vi "Tutorial.vi"() -> ()   [LabVIEW 2023]
uses:
  parametertype.ctl
  <vilib>/regexp/Match Regular Expression.xnode
  SECoP.lvlib
panel:
  in  "stop":bool
  out "log 2":string
  out "error out":errorcluster
  in  "stop 2":bool
  in  "DLL path":path=path "D:/shall-repos/SHALL-LabVIEW/64bit"
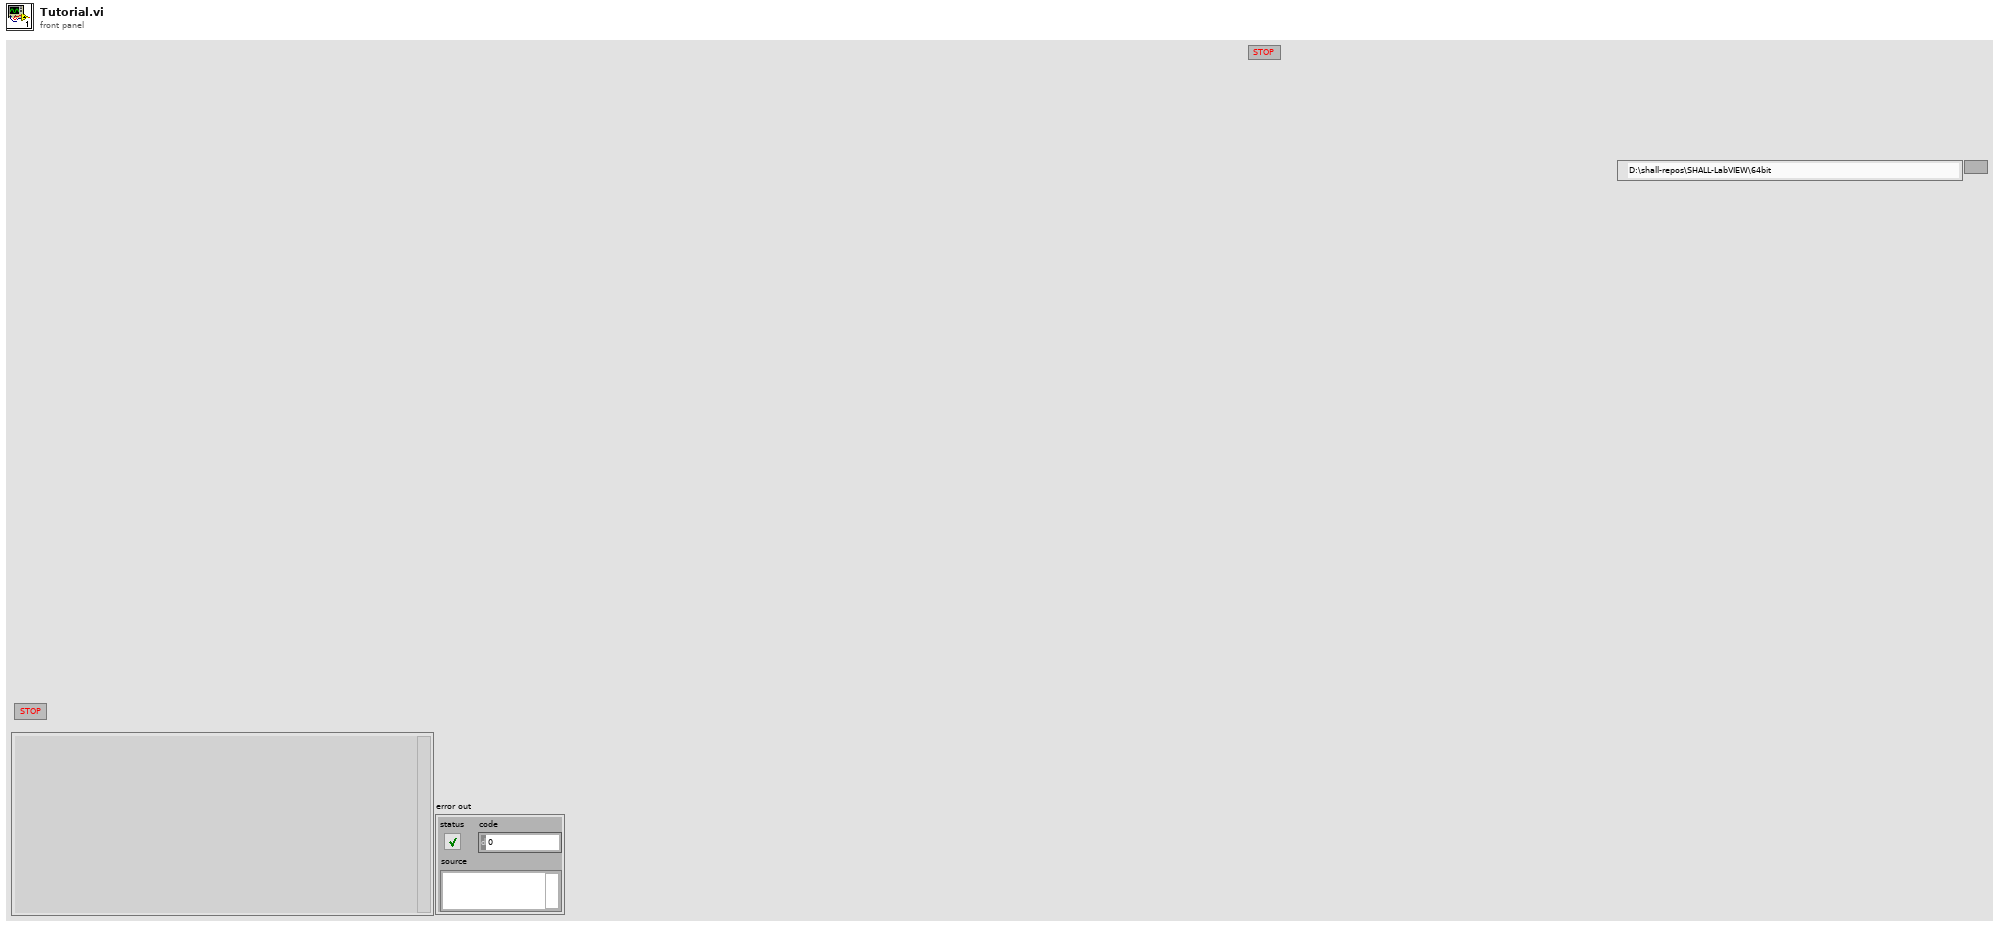
[diagram p1: front panel]
types:
  T1 = typedef "parametertype.ctl" = enum8{"readonly", "readwrite", "command"}
  T2 = cluster{"name":string, "type":T1, "datatype":string, "description":string, dbl}[]
  T3 = typedef "SECoP.lvlib/SECoP-libraries.ctl" = cluster{"serverDLL":path, "variantDLL":path, "cleanup_mode":bool, "Context_ID":string}
  T4 = typedef "SECoP.lvlib/SECoP-action.ctl" = enum32{"any action", "read", "change", "do cmd"}
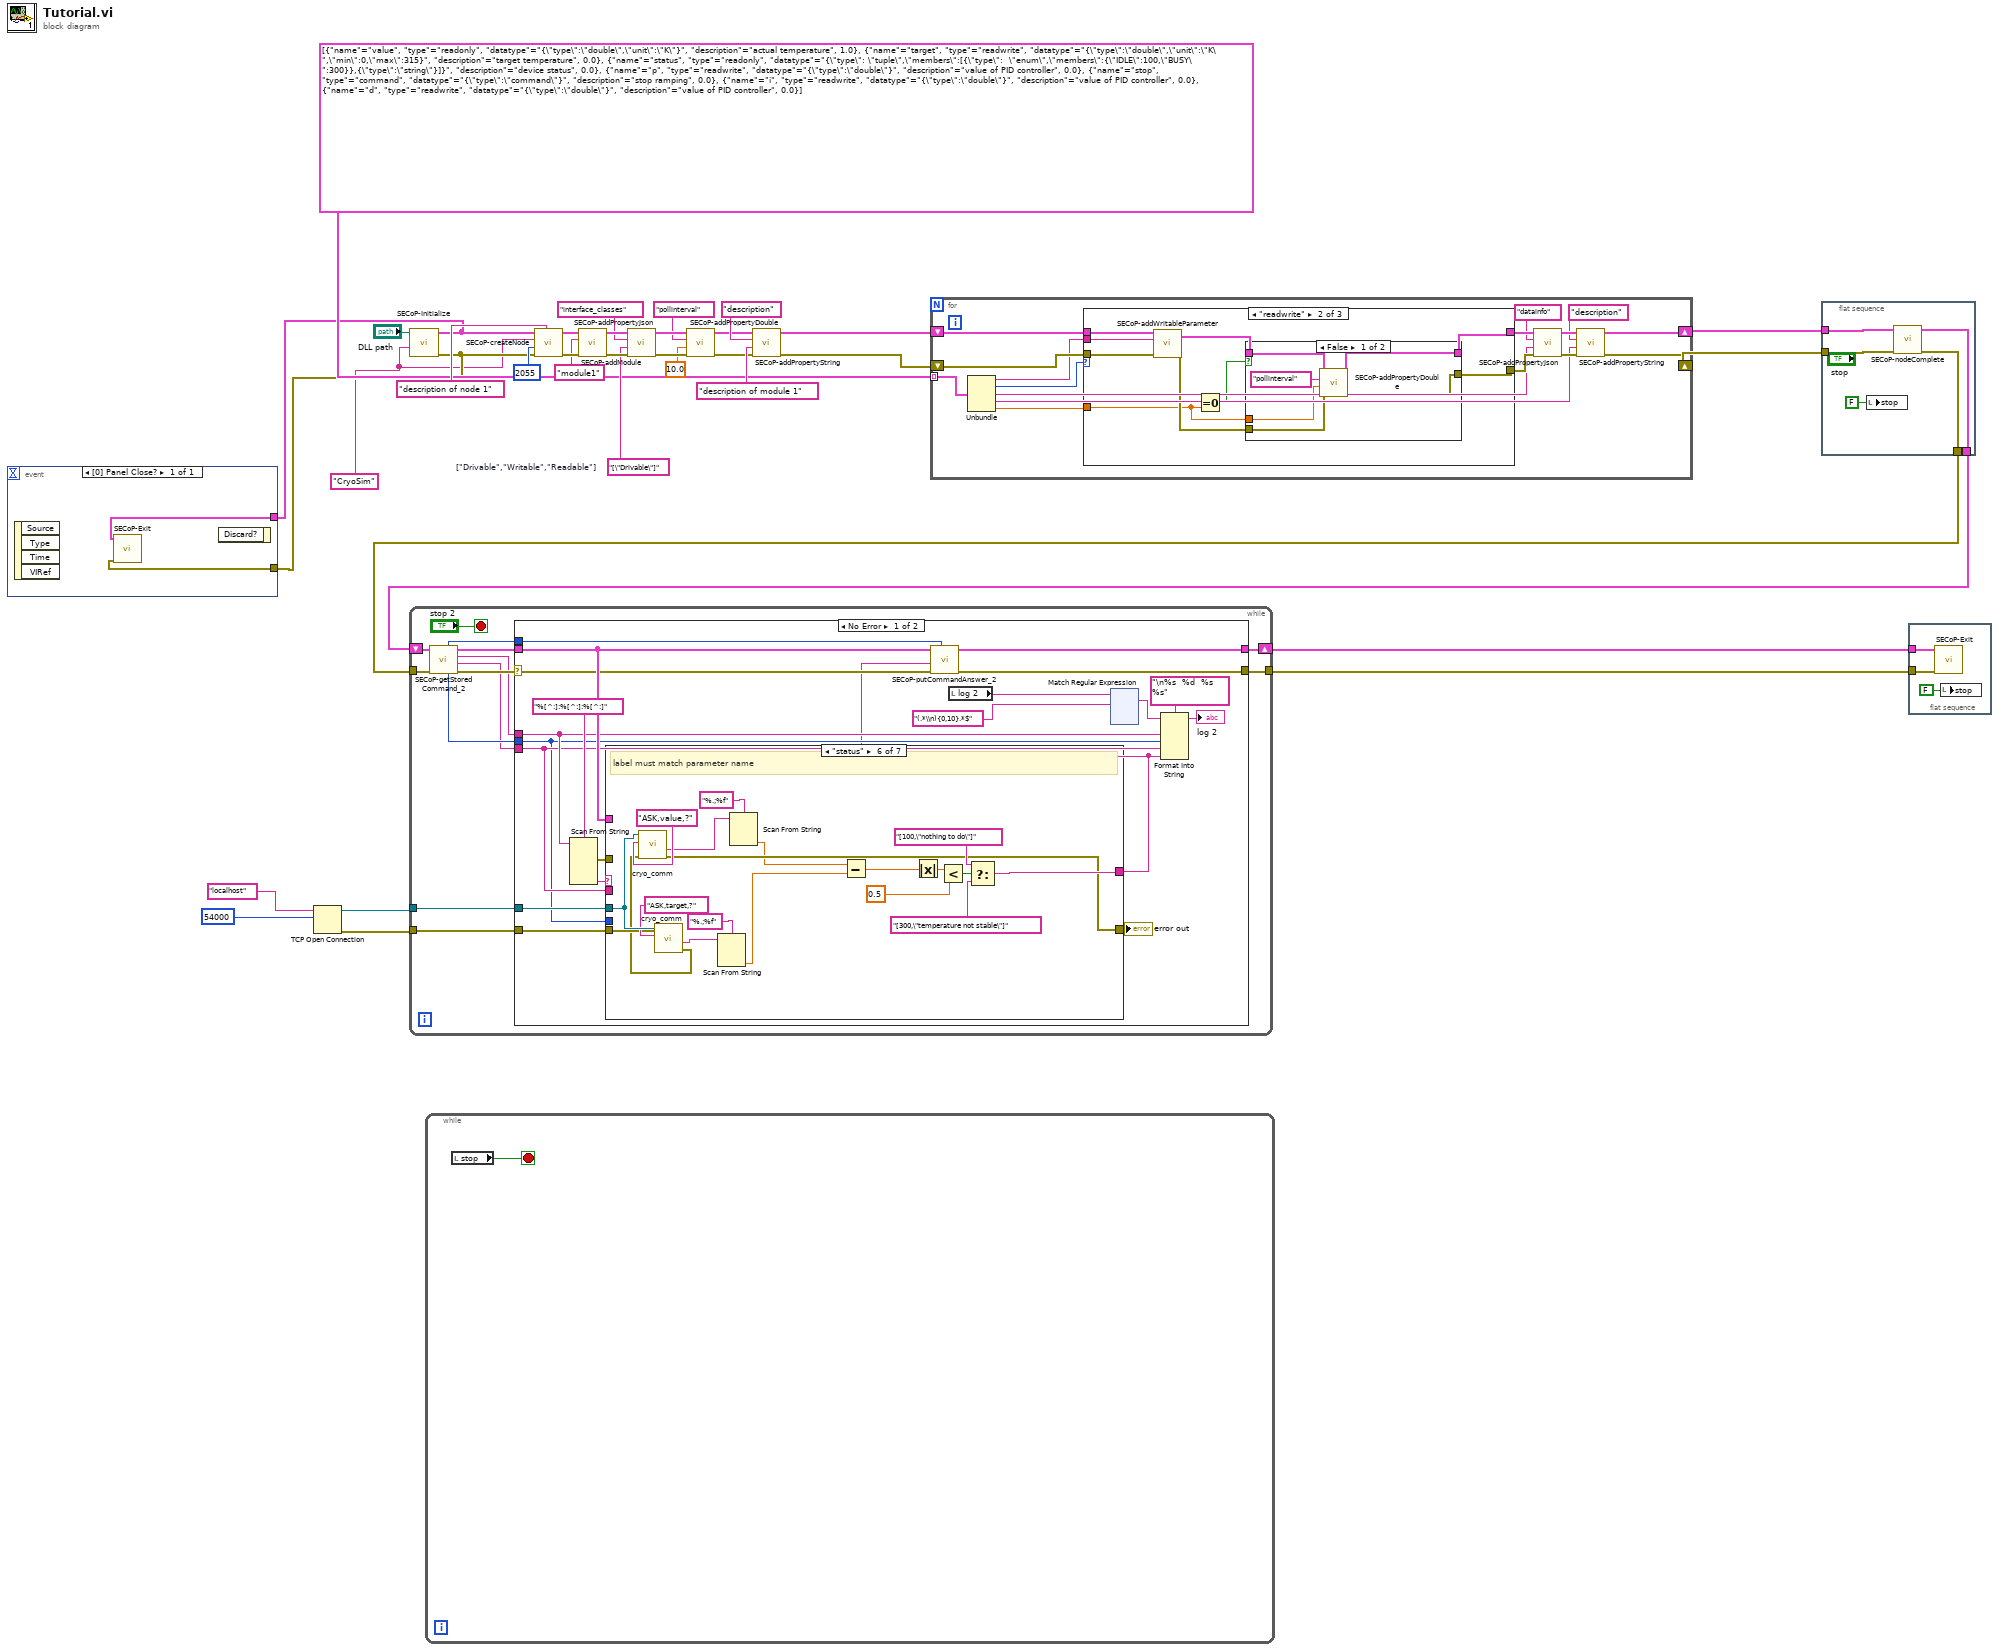
[diagram p0: block diagram]
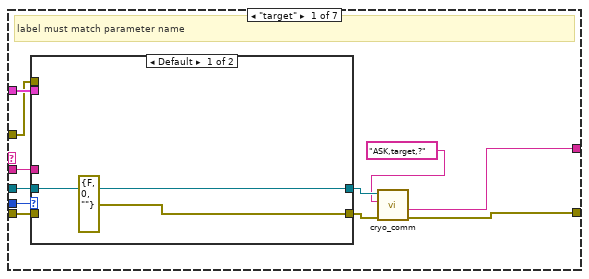
[diagram p2: hidden frame]
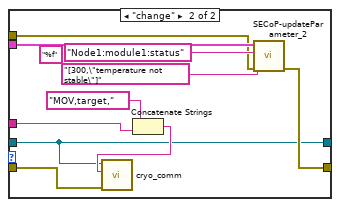
[diagram p3: hidden frame]
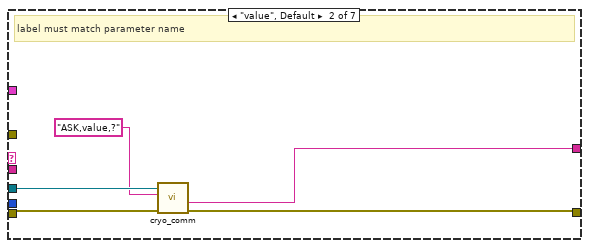
[diagram p4: hidden frame]
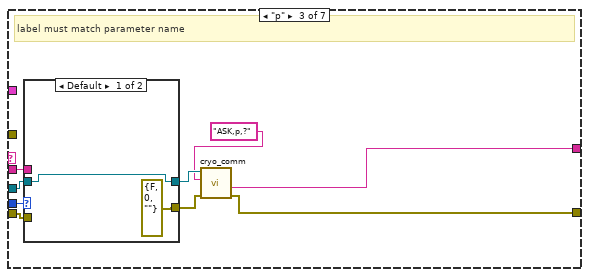
[diagram p5: hidden frame]
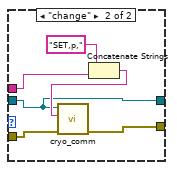
[diagram p6: hidden frame]
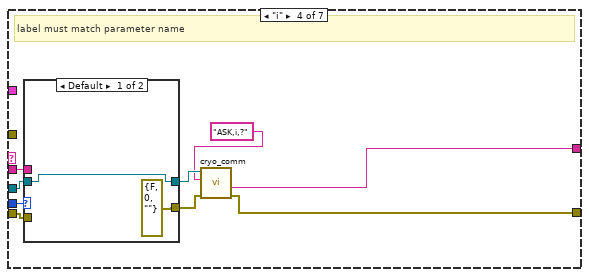
[diagram p7: hidden frame]
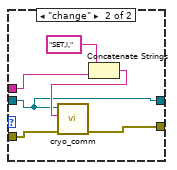
[diagram p8: hidden frame]
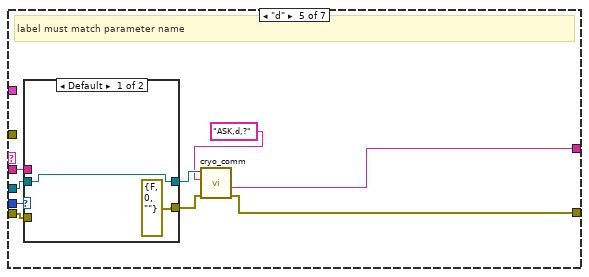
[diagram p9: hidden frame]
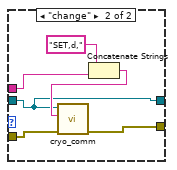
[diagram p10: hidden frame]
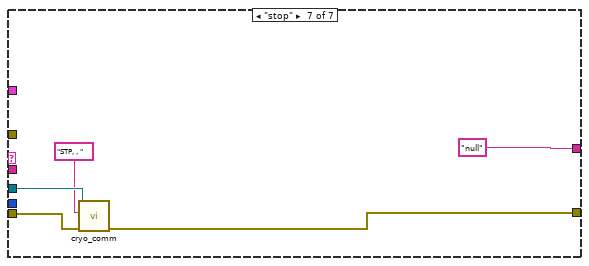
[diagram p11: hidden frame]
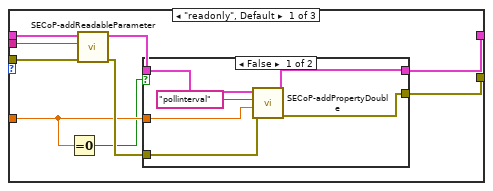
[diagram p13: hidden frame]
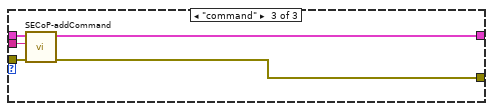
[diagram p16: hidden frame]
diagram:
  w25 = "[\"Drivable\"]"  # ["Drivable","Writable","Readable"]
  w1 = "CryoSim" ("id")
  # "description"
  # "data type as SECoP \"datainfo\""
  # "type"
  # "parameter"
  n1 = TCP Open Connection(address="localhost", remote port or service name=54000) -> (connection ID=w2:refnum<k5>, error out=w3:errorcluster)  [unwired: 3 in]
  n2 = while {
    shift-right: [w47] -> w7
    shift-left: w4 -> [w46]
    tunnel: w5 -> [w45]
    tunnel: [w38] -> w6
    tunnel: w2 -> [w36]
    tunnel: w3 -> [w35]
    stop <- "stop 2" stop-if-true
    n3 = call "SECoP-getStoredCommand_2.vi"("error in (no error)"=w45, "DLL path (in)"=w46) -> ("error out"=w43:errorcluster, "arguments/setvalue"=w39:string, "command/parameter path"=w40:string, "DLL path (out)"=w44:T3, "action"=w41:T4, "command id"=w42:u64)  [unwired: 4 in]
    n4 = case shown="No Error" w43 {
      selector: w43 -> [w66 w288]
      tunnel: w44 -> [w67 w289]
      tunnel: [w65 w289] -> w47
      tunnel: w42 -> [w64 _]
      tunnel: w40 -> [w57 _]
      tunnel: w39 -> [w53 _]
      tunnel: w41 -> [w52 _]
      tunnel: [w63 w288] -> w38
      tunnel: w36 -> [w54 _]
      tunnel: w35 -> [w50 _]
      frame No Error {
        n5 = Scan From String(format string="%[^:]:%[^:]:%[^:]", input string=w57) -> (error out=w56:errorcluster, output 3=w48:string)  [unwired: 7 in, 2 out]
        n6 = case shown="\"status\"" w48 {
          tunnel: [w71 w92 w97 w114 w131 w159 "null"] -> w49
          tunnel: w56 -> [w68 _ _ _ _ _ _]
          tunnel: w54 -> [w77 w93 w103 w120 w137 w158 w169]
          tunnel: w53 -> [w78 _ w102 w119 w136 _ _]
          tunnel: w52 -> [w76 _ w104 w121 w138 _ _]
          tunnel: [w72 w94 w98 w115 w132 w154 w166] -> w51
          tunnel: w50 -> [w75 w95 w101 w118 w135 w155 w168]
          tunnel: w67 -> [w74 _ _ _ _ _ _]
          frame "target" {
            # "label must match parameter name"
            n7 = case shown="Default" w76 {
              tunnel: w78 -> [_ w84]
              tunnel: w77 -> [w80 w82]
              tunnel: [errorcluster {"status"=FALSE, "code"=0, "source"=""} ("error out") w89] -> w73
              tunnel: [w80 w82] -> w70
              tunnel: w75 -> [_ w85]
              tunnel: w74 -> [_ w90]
              tunnel: w68 -> [_ w81]
              frame Default {
              }
              frame "change" {
                (unwired) "%f" ("format string")
                n8 = Concatenate Strings("MOV,target,", w84) -> (w83:string)
                n9 = call "cryo_comm.vi"("error in (no error)"=w85, "String"=w83, "TCP Network Connection in"=w82) -> ()  [unwired: 5 in, 4 out]
                n10 = call "SECoP-updateParameter_2.vi"("error in (no error)"=w81, "value"="[300,\"temperature not stable\"]" ("Value"), "parameter name"="Node1:module1:status" ("Parameter name"), "DLL path (in)"=w90) -> ("error out"=w89:errorcluster)  [unwired: 6 in, 1 out]
              }
            }
            n11 = call "cryo_comm.vi"("error in (no error)"=w73, "String"="ASK,target,?", "TCP Network Connection in"=w70) -> ("error out 2"=w72:errorcluster, "Message [2] (return value)"=w71:string)  [unwired: 5 in, 2 out]
          }
          frame "value", Default {
            # "label must match parameter name"
            n12 = call "cryo_comm.vi"("error in (no error)"=w95, "String"="ASK,value,?", "TCP Network Connection in"=w93) -> ("error out 2"=w94:errorcluster, "Message [2] (return value)"=w92:string)  [unwired: 5 in, 2 out]
          }
          frame "p" {
            # "label must match parameter name"
            n13 = case shown="Default" w104 {
              tunnel: w103 -> [w106 w107]
              tunnel: w102 -> [_ w109]
              tunnel: [w106 w107] -> w99
              tunnel: [errorcluster {"status"=FALSE, "code"=0, "source"=""} ("error out") w111] -> w100
              tunnel: w101 -> [_ w112]
              frame Default {
              }
              frame "change" {
                n14 = Concatenate Strings("SET,p,", w109) -> (w108:string)
                n15 = call "cryo_comm.vi"("error in (no error)"=w112, "String"=w108, "TCP Network Connection in"=w107) -> ("error out 2"=w111:errorcluster)  [unwired: 5 in, 3 out]
              }
            }
            n16 = call "cryo_comm.vi"("error in (no error)"=w100, "String"="ASK,p,?", "TCP Network Connection in"=w99) -> ("error out 2"=w98:errorcluster, "Message [2] (return value)"=w97:string)  [unwired: 5 in, 2 out]
          }
          frame "i" {
            # "label must match parameter name"
            n17 = case shown="Default" w121 {
              tunnel: w120 -> [w123 w124]
              tunnel: w119 -> [_ w126]
              tunnel: [w123 w124] -> w116
              tunnel: [errorcluster {"status"=FALSE, "code"=0, "source"=""} ("error out") w128] -> w117
              tunnel: w118 -> [_ w129]
              frame Default {
              }
              frame "change" {
                n18 = Concatenate Strings("SET,i,", w126) -> (w125:string)
                n19 = call "cryo_comm.vi"("error in (no error)"=w129, "String"=w125, "TCP Network Connection in"=w124) -> ("error out 2"=w128:errorcluster)  [unwired: 5 in, 3 out]
              }
            }
            n20 = call "cryo_comm.vi"("error in (no error)"=w117, "String"="ASK,i,?", "TCP Network Connection in"=w116) -> ("error out 2"=w115:errorcluster, "Message [2] (return value)"=w114:string)  [unwired: 5 in, 2 out]
          }
          frame "d" {
            # "label must match parameter name"
            n21 = case shown="Default" w138 {
              tunnel: w137 -> [w140 w141]
              tunnel: w136 -> [_ w143]
              tunnel: [w140 w141] -> w133
              tunnel: [errorcluster {"status"=FALSE, "code"=0, "source"=""} ("error out") w145] -> w134
              tunnel: w135 -> [_ w146]
              frame Default {
              }
              frame "change" {
                n22 = Concatenate Strings("SET,d,", w143) -> (w142:string)
                n23 = call "cryo_comm.vi"("error in (no error)"=w146, "String"=w142, "TCP Network Connection in"=w141) -> ("error out 2"=w145:errorcluster)  [unwired: 5 in, 3 out]
              }
            }
            n24 = call "cryo_comm.vi"("error in (no error)"=w134, "String"="ASK,d,?", "TCP Network Connection in"=w133) -> ("error out 2"=w132:errorcluster, "Message [2] (return value)"=w131:string)  [unwired: 5 in, 2 out]
          }
          frame "status" {
            # "label must match parameter name"
            n25 = call "cryo_comm.vi"("error in (no error)"=w155, "String"="ASK,target,?", "TCP Network Connection in"=w158) -> ("error out 2"=w153:errorcluster, "Message [2] (return value)"=w152:string)  [unwired: 5 in, 2 out]
            n26 = call "cryo_comm.vi"("error in (no error)"=w153, "String"="ASK,value,?", "TCP Network Connection in"=w158) -> ("error out 2"=w154:errorcluster, "Message [2] (return value)"=w147:string)  [unwired: 5 in, 2 out]
            n27 = Scan From String(format string="%.;%f", input string=w152) -> (output 1=w150:dbl)  [unwired: 3 in, 3 out]
            n28 = Scan From String(format string="%.;%f", input string=w147) -> (output 1=w148:dbl)  [unwired: 3 in, 3 out]
            n29 = Subtract(x=w148, y=w150) -> (x-y=w165:dbl)
            n30 = Absolute Value(x=w165) -> (abs(x)=w164:dbl)
            n31 = Less?(x=w164, y=0.5) -> (x < y?=w162:bool)
            n32 = Select(t="[100,\"nothing to do\"]", s=w162, f="[300,\"temperature not stable\"]") -> (s? t:f=w159:string)
          }
          frame "stop" {
            n33 = call "cryo_comm.vi"("error in (no error)"=w168, "String"="STP, , ", "TCP Network Connection in"=w169) -> ("error out 2"=w166:errorcluster)  [unwired: 5 in, 3 out]
          }
        }
        "error out" <- w51
        n34 = call "SECoP-putCommandAnswer_2.vi"("command id"=w64, "error in (no error)"=w66, "value"=w49, "DLL path (in)"=w67) -> ("error out"=w63:errorcluster, "DLL path (out)"=w65:T3)  [unwired: 6 in]
        n35 = local read "log 2"() -> (w60:string)
        n36 = xnode "Match Regular Expression"("input string"=w60, "regular expression"="(.*\\n){0,10}.*$") -> ("whole match"=w61:string)  [unwired: 4 in, 4 out]
        n37 = Format Into String(format string="\n%s  %d  %s  %s", initial string=w61, w57, w52, w53, w49) -> (resulting string=→"log 2":string)  [unwired: 1 in, 1 out]
      }
      frame Error {
      }
    }
  }
  n38 = call "SECoP-Initialize.vi"("Context ID (in)"=w1, "DLL path (in)"="DLL path") -> ("error out"=w12:errorcluster, "DLL path (out)"=w13:T3)  [unwired: 8 in]
  n39 = event shown="[0] Panel Close?" {
    selector: _ -> [_]
    dyn-events: _ -> [_]
    timeout: _ -> [_]
    tunnel: w13 -> [w291]
    tunnel: w12 -> [w290]
    event Panel Close? {
      n40 = event-data() -> ()  [unwired: 1 in, 4 out]
      n41 = call "SECoP-Exit.vi"("error in (no error)"=w290, "DLL path (in)"=w291) -> ()  [unwired: 9 in, 1 out]
      n42 = event-data() -> ()  [unwired: 2 in, 1 out]
    }
  }
  n43 = while {
    stop <- w292 stop-if-true
    n44 = local read "stop"() -> (w292:bool)
  }
  n45 = call "SECoP-createNode.vi"("description"="description of node 1", "error in (no error)"=w12, "TCP port"=u16 2055, "node id"=w1, "DLL path (in)"=w13) -> ("error out"=w30:errorcluster, "DLL path (out)"=w33:T3)  [unwired: 5 in]
  n46 = call "SECoP-addModule.vi"("error in (no error)"=w30, "module name"="module1" ("name"), "DLL path (in)"=w33) -> ("error out"=w27:errorcluster, "DLL path (out)"=w28:T3)  [unwired: 7 in]
  n47 = call "SECoP-addPropertyJson.vi"("error in (no error)"=w27, "property value"=w25, "property name"="interface_classes" ("name"), "DLL path (in)"=w28) -> ("error out"=w18:errorcluster, "DLL path (out)"=w20:T3)  [unwired: 6 in]
  n48 = call "SECoP-addPropertyDouble.vi"("error in (no error)"=w18, "property value"=10.0, "property name"="pollinterval", "DLL path (in)"=w20) -> ("error out"=w17:errorcluster, "DLL path (out)"=w19:T3)  [unwired: 6 in]
  n49 = call "SECoP-addPropertyString.vi"("error in (no error)"=w17, "property value"="description of module 1" ("name"), "property name"="description" ("name"), "DLL path (in)"=w19) -> ("error out"=w23:errorcluster, "DLL path (out)"=w24:T3)  [unwired: 6 in]
  n50 = for {
    tunnel: T2 [{"name"="value", "type"=enum."readonly", "datatype"="{\"type\":\"double\",\"unit\":\"K\"}", "description"="actual temperature", 1.0}, {"name"="target", "type"=enum."readwrite", "datatype"="{\"type\":\"double\",\"unit\":\"K\",\"min\":0,\"max\":315}", "description"="target temperature", 0.0}, {"name"="status", "type"=enum."readonly", "datatype"="{\"type\": \"tuple\",\"members\":[{\"type\":  \"enum\",\"members\":{\"IDLE\":100,\"BUSY\":300}},{\"type\":\"string\"}]}", "description"="device status", 0.0}, {"name"="p", "type"=enum."readwrite", "datatype"="{\"type\":\"double\"}", "description"="value of PID controller", 0.0}, {"name"="stop", "type"=enum."command", "datatype"="{\"type\":\"command\"}", "description"="stop ramping", 0.0}, {"name"="i", "type"=enum."readwrite", "datatype"="{\"type\":\"double\"}", "description"="value of PID controller", 0.0}, {"name"="d", "type"=enum."readwrite", "datatype"="{\"type\":\"double\"}", "description"="value of PID controller", 0.0}] -> [w296] mode=indexing
    shift-right: [w295] -> w11
    shift-left: w24 -> [w305]
    shift-right: [w294] -> w10
    shift-left: w23 -> [w304]
    n51 = Unbundle(w296) -> ("name"=w297:string, "type"=w306:T1, "datatype"=w298:string, "description"=w299:string, w293:dbl)
    n52 = case shown="\"readwrite\"" w306 {
      tunnel: w297 -> [w316 w334 w343]
      tunnel: w305 -> [w317 w333 w347]
      tunnel: [w312 w330 w346] -> w303
      tunnel: [w311 w328 w344] -> w302
      tunnel: w304 -> [w315 w332 w345]
      tunnel: w293 -> [w310 w326 _]
      frame "readonly", Default {
        n53 = Equal To 0?(x=w310) -> (x = 0?=w309:bool)
        n54 = call "SECoP-addReadableParameter.vi"("error in (no error)"=w315, "parameter name"=w316, "DLL path (in)"=w317) -> ("error out"=w313:errorcluster, "DLL path (out)"=w314:T3)  [unwired: 7 in]
        n55 = case shown="False" w309 {
          tunnel: w314 -> [w323 w325]
          tunnel: [w321 w325] -> w312
          tunnel: w313 -> [w322 w324]
          tunnel: [w320 w324] -> w311
          tunnel: w310 -> [w318 _]
          frame False {
            n56 = call "SECoP-addPropertyDouble.vi"("error in (no error)"=w322, "property value"=w318, "property name"="pollinterval", "DLL path (in)"=w323) -> ("error out"=w320:errorcluster, "DLL path (out)"=w321:T3)  [unwired: 6 in]
          }
          frame True {
          }
        }
      }
      frame "readwrite" {
        n57 = call "SECoP-addWritableParameter.vi"("error in (no error)"=w332, "parameter name"=w334, "DLL path (in)"=w333) -> ("error out"=w329:errorcluster, "DLL path (out)"=w331:T3)  [unwired: 7 in]
        n58 = Equal To 0?(x=w326) -> (x = 0?=w327:bool)
        n59 = case shown="False" w327 {
          tunnel: w331 -> [w340 w342]
          tunnel: [w337 w342] -> w330
          tunnel: w329 -> [w339 w341]
          tunnel: [w336 w341] -> w328
          tunnel: w326 -> [w338 _]
          frame False {
            n60 = call "SECoP-addPropertyDouble.vi"("error in (no error)"=w339, "property value"=w338, "property name"="pollinterval", "DLL path (in)"=w340) -> ("error out"=w336:errorcluster, "DLL path (out)"=w337:T3)  [unwired: 6 in]
          }
          frame True {
          }
        }
      }
      frame "command" {
        n61 = call "SECoP-addCommand.vi"("error in (no error)"=w345, "command name"=w343, "DLL path (in)"=w347) -> ("error out"=w344:errorcluster, "DLL path (out)"=w346:T3)  [unwired: 7 in]
      }
    }
    n62 = call "SECoP-addPropertyJson.vi"("error in (no error)"=w302, "property value"=w298, "property name"="datainfo" ("name"), "DLL path (in)"=w303) -> ("error out"=w307:errorcluster, "DLL path (out)"=w308:T3)  [unwired: 6 in]
    n63 = call "SECoP-addPropertyString.vi"("error in (no error)"=w307, "property value"=w299, "property name"="description" ("name"), "DLL path (in)"=w308) -> ("error out"=w294:errorcluster, "DLL path (out)"=w295:T3)  [unwired: 6 in]
  }
  n64 = flat-sequence {
    tunnel: [w351] -> w4
    tunnel: [w352] -> w5
    tunnel: w11 -> [w350]
    tunnel: w10 -> [w349]
    frame #0 {
      n65 = local write "stop"(FALSE) -> ()
      n66 = call "SECoP-nodeComplete.vi"("error in (no error)"=w349, "DLL path (in)"=w350) -> ("error out"=w352:errorcluster, "DLL path (out)"=w351:T3)  [unwired: 8 in]
    }
  }
  n67 = flat-sequence {
    tunnel: w7 -> [w354]
    tunnel: w6 -> [w353]
    frame #0 {
      n68 = call "SECoP-Exit.vi"("error in (no error)"=w353, "DLL path (in)"=w354) -> ()  [unwired: 9 in, 1 out]
      n69 = local write "stop"(FALSE) -> ()
    }
  }
